vi "Read Analogue.vi"(8 "error in (no error)":errorcluster, 11 "NI Digitizer in":refnum<class "NI Digitizer.lvclass">) -> (0 "error out":errorcluster, 2 "Waveforms":waveform(dbl)[](array[waveform]), 3 "NI Digitizer out":refnum<class "NI Digitizer.lvclass">)   [LabVIEW 2025, in "Digitizer.lvlib" / "NI Digitizer.lvclass"]
uses:
  NI Digitizer.lvclass
  NI Digitizer.lvclass/NI Digitizer.ctl
  <vilib>/Analysis/NI_AALBase.lvlib
  <vilib>/Analysis/baseanly.llb/Mean (DBL).vi
  <vilib>/DAQmx/read.llb/DAQmx Read (Analog 1D Wfm NChan NSamp).vi
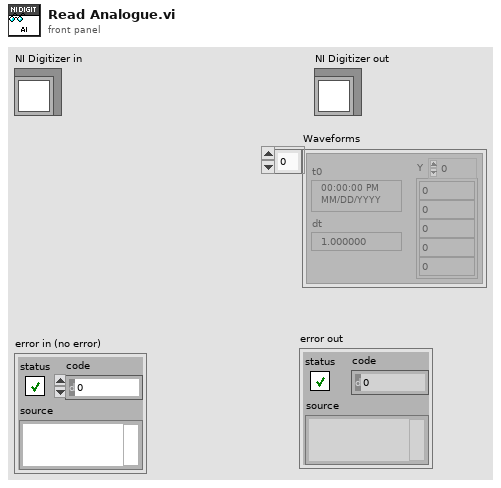
[diagram p1: front panel]
types:
  T1 = typedef "Abstract Engine.lvlibp/Abstract Instrument.lvclass/Channel.ctl" = cluster{"Alias":string, "DataType":enum16{"Anaolg Input", "Waveform"}, "Unit":enum16{"---", "V", "A", "Ohm", "Hz", "uF", "degC", "deg"}, "Upper limit":dbl, "Lower limit":dbl, "Measurement":variant}
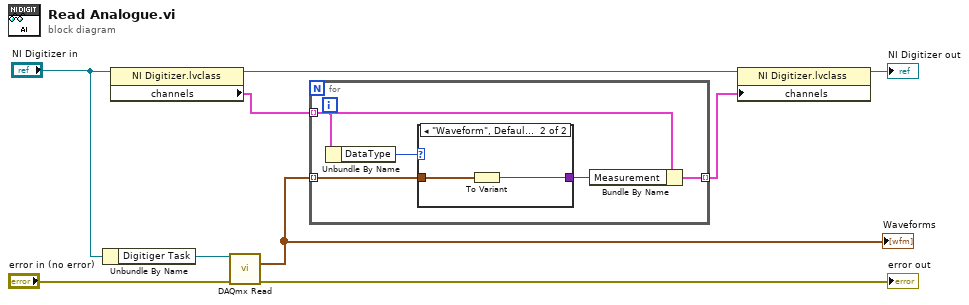
[diagram p0: block diagram]
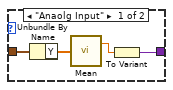
[diagram p2: hidden frame]
diagram:
  n1 = Unbundle By Name("NI Digitizer in") -> ("Digitiger Task"=w6:refnum<k21>)
  n2 = property class="NI Digitizer.lvclass"(reference="NI Digitizer in") -> (reference out=w5:refnum<class "NI Digitizer.lvclass">, "channels"=w4:T1[])  [unwired: 1 in, 1 out]
  n3 = call-poly <vilib>:"DAQmx Read.vi"("task/channels in"=w6, "error in"="error in (no error)") -> ("data"=w1:waveform(dbl)[], "error out"=→"error out":errorcluster)  [unwired: 11 in, 1 out]
  "Waveforms" <- w1
  n4 = for {
    tunnel: w1 -> [w10] mode=indexing
    tunnel: w4 -> [w11] mode=indexing
    tunnel: [w12] -> w2 mode=indexing
    n5 = Unbundle By Name(w11) -> ("DataType"=w14:enum16{"Anaolg Input", "Waveform"})
    n6 = case shown="\"Waveform\", Default" w14 {
      tunnel: w10 -> [w17 w20]
      tunnel: [w15 w19] -> w13
      frame "Anaolg Input" {
        n7 = Unbundle By Name(w17) -> ("Y"=w18:dbl[])
        n8 = call-poly <vilib>:"Mean.vi"("X"=w18) -> ("mean"=w16:dbl)  [unwired: 1 out]
        n9 = To Variant(anything=w16) -> (Variant=w15:variant)
      }
      frame "Waveform", Default {
        n10 = To Variant(anything=w20) -> (Variant=w19:variant)
      }
    }
    n11 = Bundle By Name(cluster=w11, "Measurement"=w13) -> (w12:T1)
  }
  n12 = property class="NI Digitizer.lvclass"(reference=w5, "channels"=w2) -> (reference out=→"NI Digitizer out":refnum<class "NI Digitizer.lvclass">)  [unwired: 1 in, 1 out]
